vi "append data.vi"(8 "error in (no error)":errorcluster, 9 "Array":dbl[](array[numeric]), 10 "Time Stamp":timestamp, 11 "Data Log in":refnum<class "Data Log.lvclass">) -> (0 "error out":errorcluster, 3 "Data Log out":refnum<class "Data Log.lvclass">)   [LabVIEW 2025, in "Data Log.lvclass"]
uses:
  Data Log.lvclass
  Data Log.lvclass/Data Log.ctl
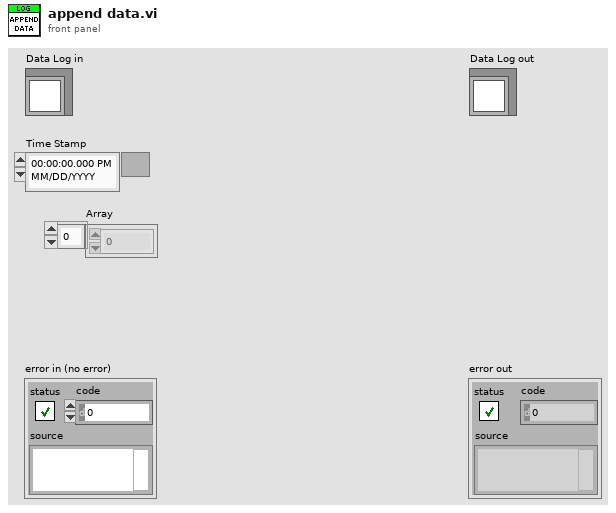
[diagram p1: front panel]
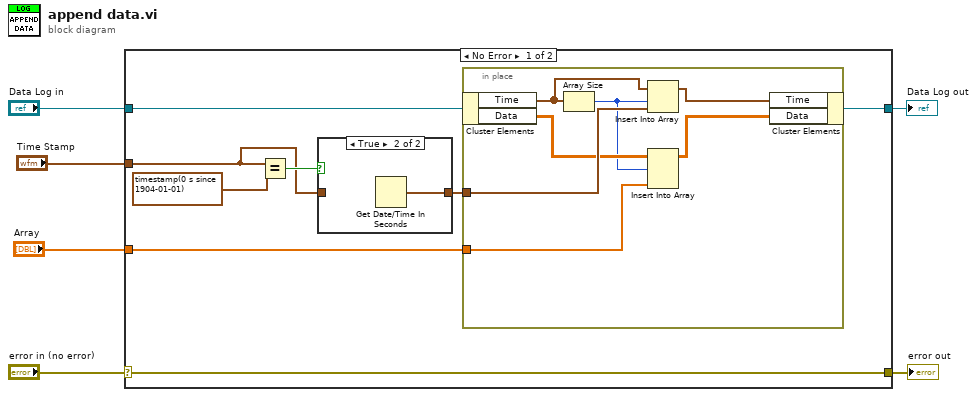
[diagram p0: block diagram]
diagram:
  n1 = case shown="No Error" "error in (no error)" {
    selector: "error in (no error)" -> [w14 w25]
    tunnel: [w14 w25] -> w5
    tunnel: [w7 w24] -> w3
    tunnel: "Data Log in" -> [w10 w24]
    tunnel: "Time Stamp" -> [w11 _]
    tunnel: "Array" -> [w8 _]
    frame No Error {
      n2 = Equal?(x=w11, y=timestamp(0 s since 1904-01-01)) -> (x = y?=w13:bool)
      n3 = case shown="True" w13 {
        tunnel: [w22 w23] -> w9
        tunnel: w11 -> [w22 _]
        frame False {
        }
        frame True {
          n4 = Get Date/Time In Seconds() -> (seconds since 1Jan1904=w23:timestamp)
        }
      }
      n5 = in-place {
        in-place-border: w9 -> [w20]
        in-place-border: w8 -> [w16]
        n6 = in-place-cluster #1(w10) -> ("Time"=w21:timestamp[], "Data"=w18:dbl[][])
        n7 = Array Size(array=w21) -> (size(s)=w17:i32)
        n8 = Insert Into Array(array=w21, index=w17, new element=w20) -> (w19:timestamp[])
        n9 = Insert Into Array(array=w18, index (row)=w17, new element=w16) -> (w15:dbl[][])  [unwired: 1 in]
        n10 = in-place-cluster #1("Time"=w19, "Data"=w15) -> (w7:refnum<class "Data Log.lvclass">)
      }
    }
    frame Error {
    }
  }
  "error out" <- w5
  "Data Log out" <- w3
